vi "strings_two_segments.vi"   [LabVIEW 2010]
types:
  T1 = enum16{"open", "open or create", "create or replace", "create", "open (read-only)"}
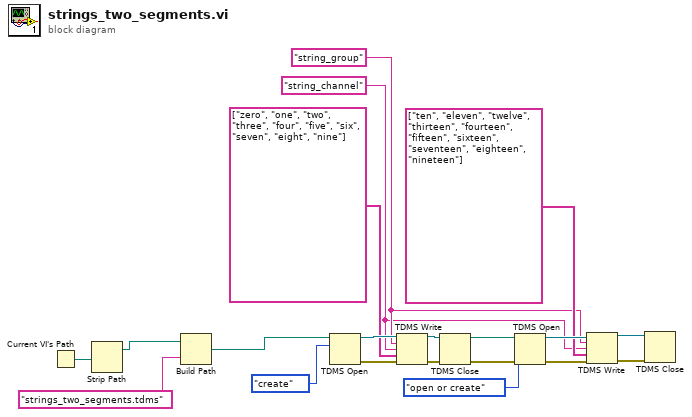
[diagram p0: block diagram]
diagram:
  w3 = "string_channel" ("channel name(s) in (Untitled)")
  w4 = "string_group" ("group name in (Untitled)")
  n1 = Current VI's Path() -> (path=w14:path)
  n2 = Strip Path(path=w14) -> (stripped path=w13:path)  [unwired: 1 out]
  n3 = Build Path(base path=w13, name or relative path="strings_two_segments.tdms") -> (appended path=w11:path)
  n4 = TDMS Open(10:T1."create" ("operation (0:open)"), 11:w11) -> (0:w20:errorcluster, 3:w19:refnum<k34>)  [unwired: 4 in]
  n5 = TDMS Write(0:w19, 5:w4, 7:w3, 9:string[] ["zero", "one", "two", "three", "four", "five", "six", "seven", "eight", "nine"] ("channel name(s) in (Untitled)"), 11:w20) -> (4:w16:refnum<k34>, 15:w15:errorcluster)  [unwired: 1 in, 2 out]
  n6 = TDMS Close(8:w15, 11:w16) -> (0:w8:errorcluster, 3:w10:path)
  n7 = TDMS Open(8:w8, 10:T1."open or create" ("operation (0:open)"), 11:w10) -> (0:w7:errorcluster, 3:w6:refnum<k34>)  [unwired: 3 in]
  n8 = TDMS Write(0:w6, 5:w4, 7:w3, 9:string[] ["ten", "eleven", "twelve", "thirteen", "fourteen", "fifteen", "sixteen", "seventeen", "eighteen", "nineteen"] ("channel name(s) in (Untitled)"), 11:w7) -> (4:w1:refnum<k34>, 15:w2:errorcluster)  [unwired: 1 in, 2 out]
  n9 = TDMS Close(8:w2, 11:w1) -> ()  [unwired: 2 out]
